vi "Facade.vi"(0 "Data In":T4, 2 "Display State In":T2, 3 "Container State":T3) -> (6 "Data Out":T4, 7 "Display State Out":T2, 8 "Action":T1)   [LabVIEW 2010, in "password.xctl"]
uses:
  password.xctl
  controls/Data.ctl
  <vilib>/_xctls/Container State.ctl
  controls/State.ctl
  <vilib>/_xctls/Action.ctl
  controls/Cluster.ctl
  <vilib>/event_ctls.llb/eventvkey.ctl
  <vilib>/_xctls/XControlSupport.lvlib
panel:
  in  "display":string
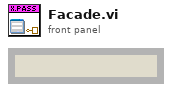
[diagram p1: front panel]
types:
  T1 = typedef "XControlSupport.lvlib/Action.ctl" = cluster{"Data Changed?":bool, "State Changed?":bool, "Action Name":string}
  T2 = typedef "password.xctl/State.ctl" = cluster{"Numeric":dbl}
  T3 = typedef "XControlSupport.lvlib/Container State.ctl" = cluster{"Indicator?":bool, "Run Mode?":bool, " Refnum":refnum<vi>}
  T4 = typedef "password.xctl/Data.ctl" = string
  T5 = enum8{"Enabled", "Disabled", "Disabled and Grayed Out"}
  T6 = typedef "eventvkey.ctl" = enum16{"ASCII", "Enter", "Return", "Shift", "Ctrl", "Alt", "Cmd", "Opt", "Caps", "NumLock", "Clear", "Break", "Up", "Down", "Left", "Right", "Insert", "Delete", "Home", "End", "PageUp", "PageDown", "Escape", "Help", "Pause", "ScrollLock", "F1", "F2", "F3", "F4", "F5", "F6", "F7", "F8", "F9", "F10", "F11", "F12", "F13", "F14", "F15", "F16", "F17", "F18", "F19", "F20", "F21", "F22", "F23", "F24", "Play", "VolumeUp", "VolumeDown", "Mute", "Two Byte Char"}
  T7 = typedef "password.xctl/Cluster.ctl" = cluster{"password":string, "display":string, "length":i32}
  T8 = typedef "Events.ctl" = enum16{"first car", "add car", "remove car", "bad change", "no change"}
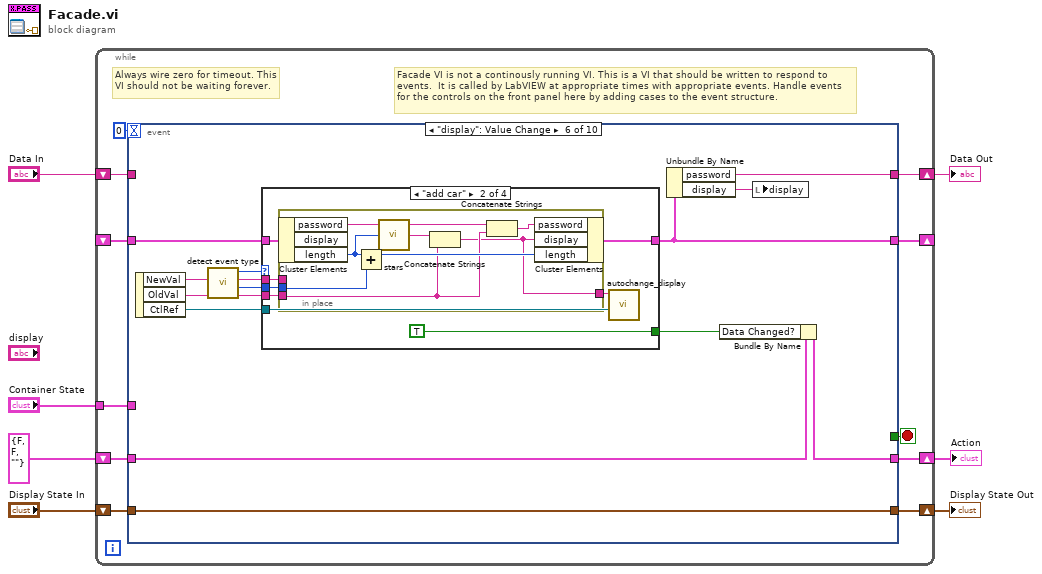
[diagram p0: block diagram]
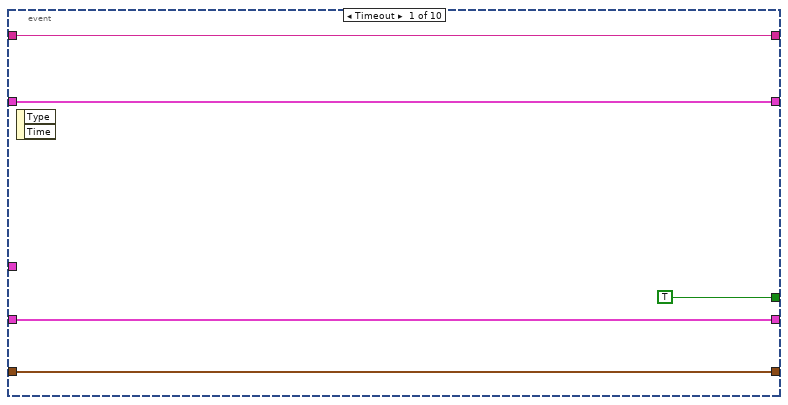
[diagram p2: hidden frame]
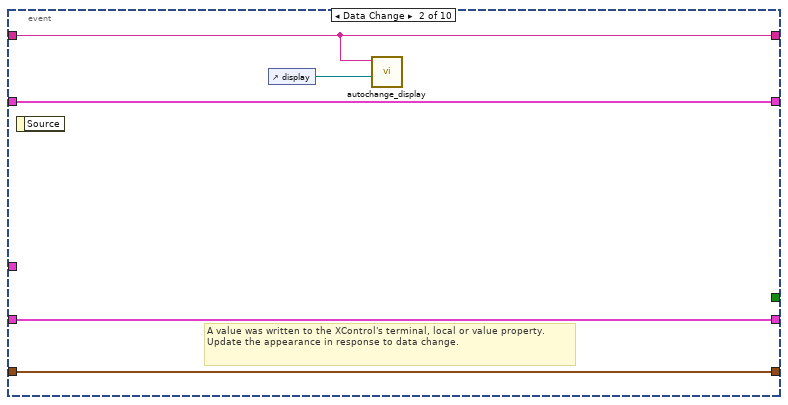
[diagram p3: hidden frame]
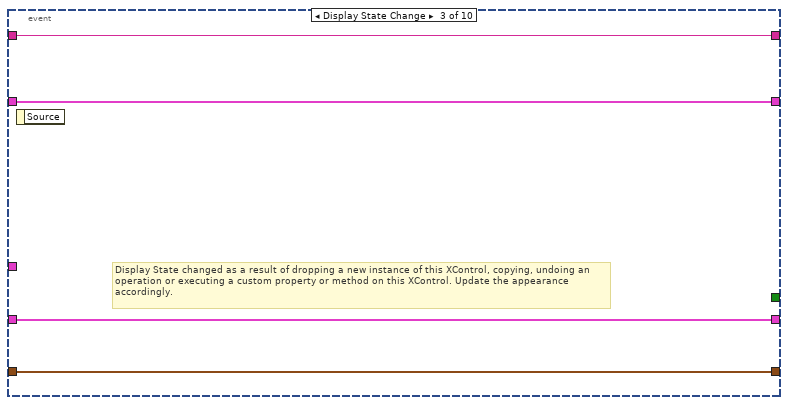
[diagram p4: hidden frame]
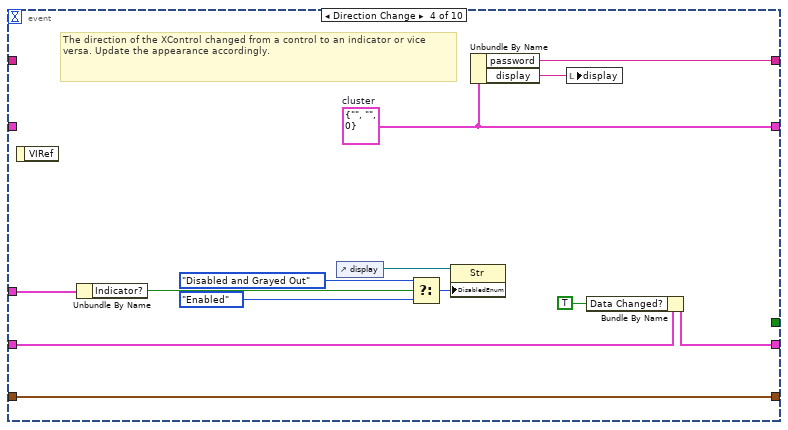
[diagram p5: hidden frame]
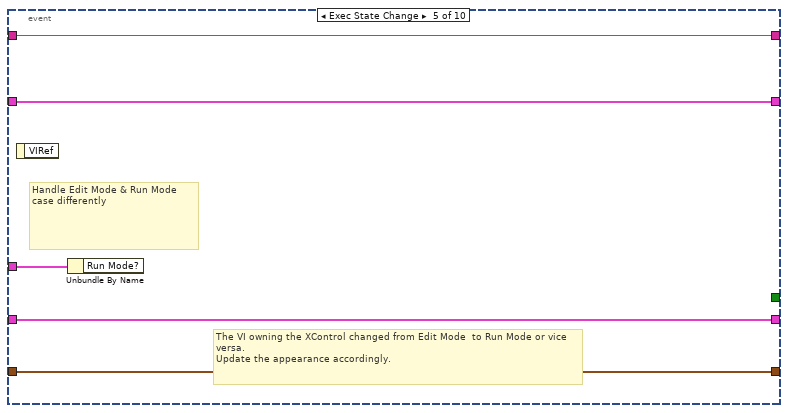
[diagram p6: hidden frame]
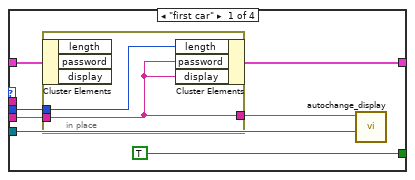
[diagram p7: hidden frame]
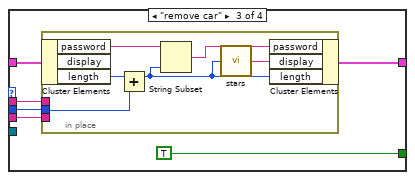
[diagram p8: hidden frame]
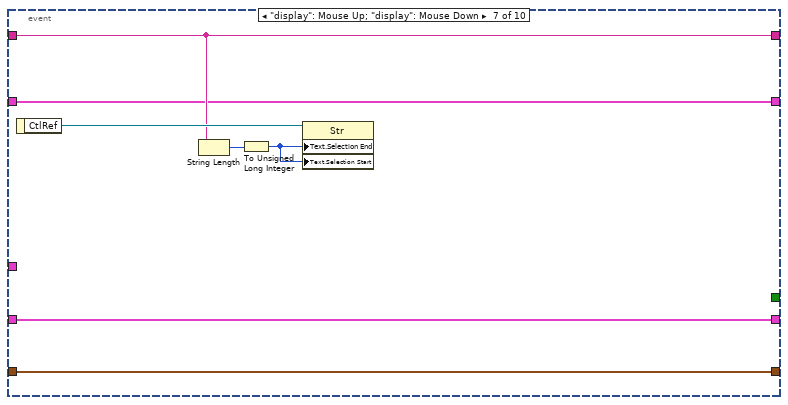
[diagram p10: hidden frame]
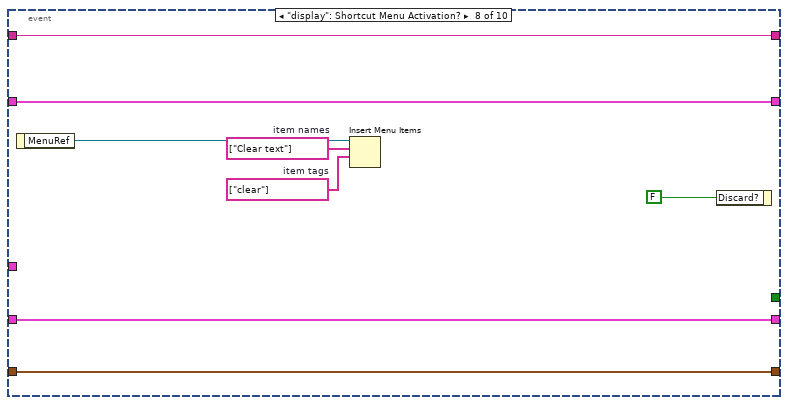
[diagram p11: hidden frame]
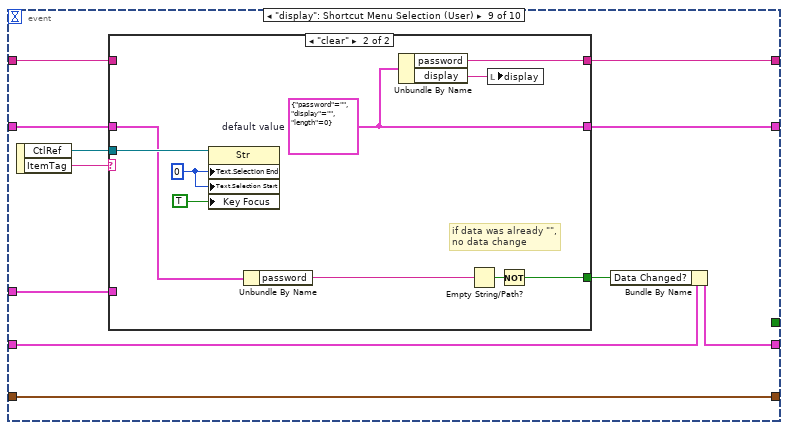
[diagram p12: hidden frame]
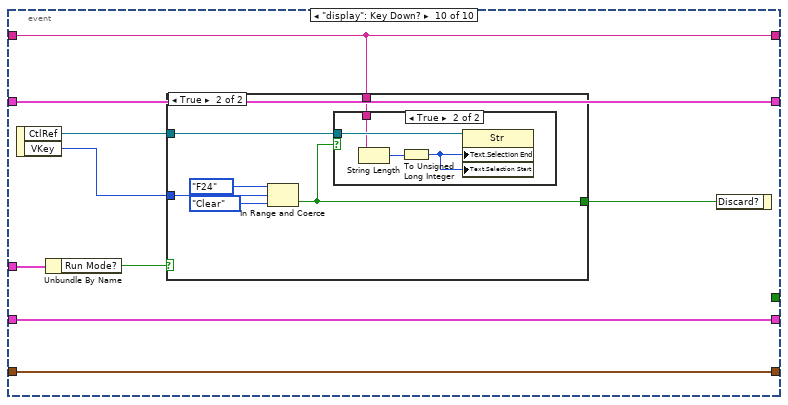
[diagram p14: hidden frame]
diagram:
  n1 = while {
    shift-right: [w17] -> w4
    shift-left: "Display State In" -> [w18]
    tunnel: "Container State" -> [w14]
    shift-right: [w12] -> w7
    shift-left: "Data In" -> [w13]
    shift-right: [w10] -> w2
    shift-left: T1 {"Data Changed?"=FALSE, "State Changed?"=FALSE, "Action Name"=""} ("Action") -> [w11]
    shift-right: [w8] -> _
    shift-left: _ -> [w9]
    stop <- w16 stop-if-true
    # "Facade VI is not a continously running VI. This is a VI that should be written to respond to events.  It is called by LabVIEW at appropriate times with appropriate events. Handle events for the controls on the front panel here by adding cases to the event structure."
    # "Always wire zero for timeout. This\nVI should not be waiting forever."
    n2 = event shown="[5] \"display\": Value Change" {
      selector: _ -> [_ _ _ _ _ _ _ _ _ _]
      dyn-events: _ -> [_ _ _ _ _ _ _ _ _ _]
      timeout: 0 -> [_ _ _ _ _ _ _ _ _ _]
      tunnel: w18 -> [w21 w28 w32 w44 w50 w65 w106 w116 w129 w147]
      tunnel: [w21 w28 w32 w44 w50 w65 w106 w116 w129 w147] -> w17
      tunnel: [TRUE _ _ _ _ _ _ _ _ _] -> w16
      tunnel: w14 -> [_ _ _ w45 w47 _ _ _ w128 w143]
      tunnel: w13 -> [w20 w25 w31 _ w46 _ w108 w118 w125 w149]
      tunnel: [w20 w25 w31 w37 w46 w54 w108 w118 w126 w149] -> w12
      tunnel: [w22 w27 w30 w34 w49 w58 w107 w117 w123 w148] -> w10
      tunnel: w11 -> [w22 w27 w30 w35 w49 w59 w107 w117 w124 w148]
      tunnel: [w19 w26 w29 w38 w48 w55 w104 w115 w121 w144] -> w8
      tunnel: w9 -> [w19 w26 w29 _ w48 w62 w104 w115 w120 w144]
      event Timeout {
        n3 = event-data() -> ()  [unwired: 1 in, 2 out]
      }
      event Data Change {
        # "A value was written to the XControl's terminal, local or value property.\nUpdate the appearance in response to data change."
        n4 = event-data() -> ()  [unwired: 1 in, 1 out]
        n5 = control-ref of="display"() -> (w24:refnum<vi>)
        n6 = call "autochange_display.vi"("display ref"=w24, "new val"=w25) -> ()  [unwired: 10 in]
      }
      event Display State Change {
        # "Display State changed as a result of dropping a new instance of this XControl, copying, undoing an operation or executing a custom property or method on this XControl. Update the appearance accordingly."
        n7 = event-data() -> ()  [unwired: 1 in, 1 out]
      }
      event Direction Change {
        w38 = T7 {"password"="", "display"="", "length"=0}  # cluster
        # "The direction of the XControl changed from a control to an indicator or vice versa. Update the appearance accordingly."
        n8 = event-data() -> ()  [unwired: 1 in, 1 out]
        n9 = Unbundle By Name(w45) -> ("Indicator?"=w41:bool)
        n10 = control-ref of="display"() -> (w43:refnum<vi>)
        n11 = Select(t=T5."Disabled and Grayed Out", s=w41, f=T5."Enabled") -> (s? t:f=w42:T5)
        n12 = property class="Str"(reference=w43, "DisabledEnum"=w42) -> ()  [unwired: 1 in, 2 out]
        n13 = Unbundle By Name(w38) -> ("password"=w37:string, "display"=w36:string)
        n14 = local write "display"(w36) -> ()
        n15 = Bundle By Name(cluster=w35, "Data Changed?"=TRUE) -> (w34:T1)
      }
      event Exec State Change {
        # "The VI owning the XControl changed from Edit Mode  to Run Mode or vice versa.\nUpdate the appearance accordingly."
        # "Handle Edit Mode & Run Mode\ncase differently"
        n16 = event-data() -> ()  [unwired: 1 in, 1 out]
        n17 = Unbundle By Name(w47) -> ()  [unwired: 1 out]
      }
      event "display": Value Change {
        n18 = event-data() -> ("NewVal"=w64:string, "OldVal"=w63:string, "CtlRef"=w51:refnum<vi>)  [unwired: 1 in]
        n19 = call "detect event type.vi"("OldVal"=w63, "NewVal"=w64) -> ("diff"=w60:string, "#"=w61:i32, "NewVal dup"=w56:string, "event"=w53:T8)  [unwired: 4 in]
        n20 = case shown="\"add car\"" w53 {
          tunnel: w62 -> [w72 w82 w96 w103]
          tunnel: w61 -> [w71 w81 w95 _]
          tunnel: w60 -> [w70 w80 w94 _]
          tunnel: [TRUE TRUE TRUE _] -> w57
          tunnel: w56 -> [_ w77 w91 _]
          tunnel: [w68 w78 w92 w103] -> w55
          tunnel: w51 -> [w66 w76 _ _]
          frame "first car" {
            n21 = in-place {
              in-place-border: w71 -> [w74]
              in-place-border: w70 -> [w73]
              in-place-border: [w73] -> w67
              n22 = in-place-cluster #1(w72) -> ()  [unwired: 3 out]
              n23 = in-place-cluster #1("length"=w74, "password"=w73, "display"=w73) -> (w68:T7)
            }
            n24 = call "autochange_display.vi"("display ref"=w66, "new val"=w67) -> ()  [unwired: 10 in]
          }
          frame "add car" {
            n25 = in-place {
              in-place-border: w81 -> [w90]
              in-place-border: w80 -> [w84]
              in-place-border: w77 -> [_]
              in-place-border: [w83] -> w75
              n26 = in-place-cluster #2(w82) -> ("password"=w88:string, "length"=w86:i32)  [unwired: 1 out]
              n27 = Add(x=w86, y=w90) -> (x+y=w89:i32)
              n28 = call "stars.vi"("n"=w86) -> ("n stars"=w85:string)
              n29 = Concatenate Strings(w85, w84) -> (w83:string)
              n30 = Concatenate Strings(w88, w84) -> (w87:string)
              n31 = in-place-cluster #2("password"=w87, "display"=w83, "length"=w89) -> (w78:T7)
            }
            n32 = call "autochange_display.vi"("display ref"=w76, "new val"=w75) -> ()  [unwired: 10 in]
          }
          frame "remove car" {
            n33 = in-place {
              in-place-border: w95 -> [w102]
              in-place-border: w94 -> [_]
              in-place-border: w91 -> [_]
              n34 = in-place-cluster #3(w96) -> ("password"=w98:string, "length"=w101:i32)  [unwired: 1 out]
              n35 = Add(x=w101, y=w102) -> (x+y=w99:i32)
              n36 = String Subset(string=w98, length (rest)=w99) -> (substring=w97:string)  [unwired: 1 in]
              n37 = call "stars.vi"("n"=w99) -> ("n stars"=w100:string)
              n38 = in-place-cluster #3("password"=w97, "display"=w100, "length"=w99) -> (w92:T7)
            }
          }
          frame Default {
          }
        }
        n39 = Unbundle By Name(w55) -> ("password"=w54:string, "display"=w52:string)
        n40 = Bundle By Name(cluster=w59, "Data Changed?"=w57) -> (w58:T1)
        n41 = local write "display"(w52) -> ()
      }
      event "display": Mouse Up; "display": Mouse Down {
        n42 = event-data() -> ("CtlRef"=w110:refnum<vi>)  [unwired: 1 in]
        n43 = String Length(string=w108) -> (length=w109:i32)
        n44 = To Unsigned Long Integer(number=w109) -> (unsigned 32bit integer=w105:u32)
        n45 = property class="Str"(reference=w110, "Text.Selection End"=w105, "Text.Selection Start"=w105) -> ()  [unwired: 1 in, 2 out]
      }
      event "display": Shortcut Menu Activation? {
        w112 = string[] ["clear"]  # item tags
        w113 = string[] ["Clear text"]  # item names
        n46 = event-data() -> ("MenuRef"=w114:refnum<k9>)  [unwired: 1 in]
        n47 = Insert Menu Items(7:w112, 8:w113, 9:w114) -> ()  [unwired: 3 in, 3 out]
        n48 = event-data("Discard?"=FALSE) -> ()  [unwired: 1 in, 1 out]
      }
      event "display": Shortcut Menu Selection (User) {
        n49 = event-data() -> ("CtlRef"=w119:refnum<vi>, "ItemTag"=w127:string)  [unwired: 1 in]
        n50 = case shown="\"clear\"" w127 {
          tunnel: w128 -> [_ _]
          tunnel: [w131 w139] -> w126
          tunnel: w125 -> [w131 _]
          tunnel: [_ w137] -> w122
          tunnel: [w130 w141] -> w121
          tunnel: w120 -> [w130 w134]
          tunnel: w119 -> [_ w135]
          frame Default {
          }
          frame "clear" {
            w136 = u32 0
            w141 = T7 {"password"="", "display"="", "length"=0}  # default value
            # "if data was already \"\",\nno data change"
            n51 = property class="Str"(reference=w135, "Text.Selection End"=w136, "Text.Selection Start"=w136, "Key Focus"=TRUE) -> ()  [unwired: 1 in, 2 out]
            n52 = Unbundle By Name(w134) -> ("password"=w133:string)
            n53 = Unbundle By Name(w141) -> ("password"=w139:string, "display"=w140:string)
            n54 = Empty String/Path?(string/path=w133) -> (empty?=w138:bool)
            n55 = local write "display"(w140) -> ()
            n56 = Not(x=w138) -> (.not. x?=w137:bool)
          }
        }
        n57 = Bundle By Name(cluster=w124, "Data Changed?"=w122) -> (w123:T1)
      }
      event "display": Key Down? {
        n58 = event-data() -> ("CtlRef"=w150:refnum<vi>, "VKey"=w146:T6)  [unwired: 1 in]
        n59 = Unbundle By Name(w143) -> ("Run Mode?"=w142:bool)
        n60 = case shown="True" w142 {
          tunnel: w150 -> [_ w156]
          tunnel: w149 -> [_ w155]
          tunnel: w146 -> [_ w152]
          tunnel: [_ w151] -> w145
          frame False {
          }
          frame True {
            n61 = In Range and Coerce(upper limit=eventvkey."F24", x=w152, lower limit=eventvkey."Clear") -> (In Range?=w151:bool)  [unwired: 1 out]
            n62 = case shown="True" w151 {
              tunnel: w156 -> [_ w160]
              tunnel: w155 -> [_ w158]
              frame False {
              }
              frame True {
                n63 = String Length(string=w158) -> (length=w159:i32)
                n64 = To Unsigned Long Integer(number=w159) -> (unsigned 32bit integer=w157:u32)
                n65 = property class="Str"(reference=w160, "Text.Selection End"=w157, "Text.Selection Start"=w157) -> ()  [unwired: 1 in, 2 out]
              }
            }
          }
        }
        n66 = event-data("Discard?"=w145) -> ()  [unwired: 1 in, 1 out]
      }
    }
  }
  "Display State Out" <- w4
  "Data Out" <- w7
  "Action" <- w2
